vi "Create VI By Template (Replace Control).vi"(8 "error in":errorcluster, 9 "Control Replacement Params":T1[](array[typedef])=[{"Placeholder Name"="PK", "CTL File Path"=path "C:/Users/OneEd/OneDrive/Desktop/MicroPort Job/CTDB/src/db_script/PK Test.ctl", "Indicator"=FALSE}, {"Placeholder Name"="Data", "CTL File Path"=path "C:/Users/OneEd/OneDrive/Desktop/MicroPort Job/CTDB/src/db_script/Value Test.ctl", "Indicator"=TRUE}], 10 "Save as":path=path "C:/Users/OneEd/OneDrive/Desktop/MicroPort Job/CTDB/src/sql_function/DB Select Template.vi", 11 "Template VI Path":path=path "C:/Users/OneEd/OneDrive/Desktop/MicroPort Job/CTDB/src/db_script/DB Select Template.vi") -> (0 "error out":errorcluster, 3 "Save as out":path=path "C:/Users/OneEd/OneDrive/Desktop/MicroPort Job/CTDB/src/db_script/DB Select Template.vi")   [LabVIEW 2022 SP3, in "EDT VI Script.lvlib"]
uses:
  EDT VI Script.lvlib
  Control Replacement Param.ctl
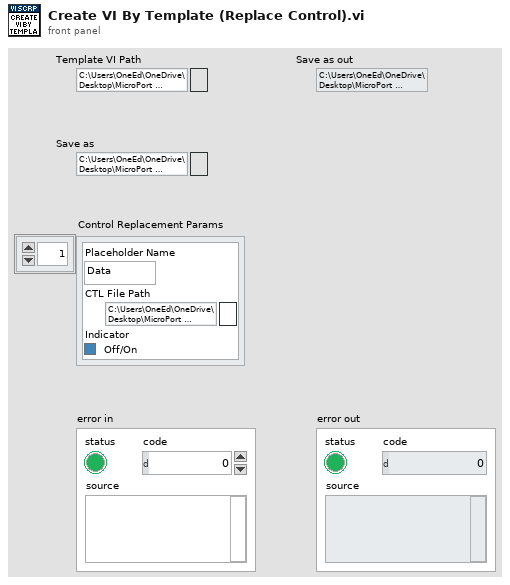
[diagram p1: front panel]
types:
  T1 = typedef "EDT VI Script.lvlib/Control Replacement Param.ctl" = cluster{"Placeholder Name":string, "CTL File Path":path, "Indicator":bool}
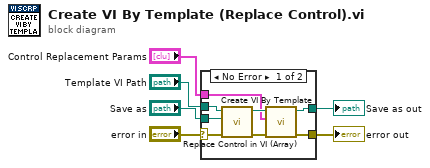
[diagram p0: block diagram]
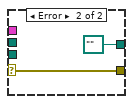
[diagram p2: hidden frame]
diagram:
  n1 = case shown="No Error" "error in" {
    selector: "error in" -> [w11 w16]
    tunnel: [w8 w16] -> w5
    tunnel: "Template VI Path" -> [w14 _]
    tunnel: "Control Replacement Params" -> [w7 _]
    tunnel: [w9 path "" ("Path")] -> w2
    tunnel: "Save as" -> [w13 _]
    frame No Error {
      n2 = call "Create VI By Template.vi"("error in"=w11, "Template VI Path"=w13, "Save as"=w14) -> ("error out"=w10:errorcluster, "Save as out"=w12:path)  [unwired: 7 in]
      n3 = call "Replace Control in VI (Array).vi"("error in"=w10, "Control Replacement Params"=w7, "Original VI"=w12) -> ("error out"=w8:errorcluster, "Save as out"=w9:path)  [unwired: 7 in]
    }
    frame Error {
    }
  }
  "error out" <- w5
  "Save as out" <- w2
